vi "Get Tweets Search New.vi"(8 "error in":errorcluster, 9 "Tweets to Read (10)":i32=10 min=0 max=200 step=1, 10 "Query":string="#LVHacker", 11 "Twitter Handle In":T1={"OAuth Credentials"={"Signature Method"=enum."HMAC-SHA1", "Version"="1.0", "Client"={"Token"="", "Secret"=""}, "Access"={"Token"="", "Secret"=""}}, "since ID"="", "max ID"="", "Screen Name"=""}) -> (0 "error out":errorcluster, 1 "Actual Num of Tweets Read":i32, 2 "New Tweets Read":T5[](array[typedef]), 3 "Twitter Handle Out":T1={"OAuth Credentials"={"Signature Method"=enum."HMAC-SHA1", "Version"="1.0", "Client"={"Token"="", "Secret"=""}, "Access"={"Token"="", "Secret"=""}}, "since ID"="", "max ID"="", "Screen Name"=""}, 5 "Time Stamp of Newest Tweet":timestamp)   [LabVIEW 2011, in "i3-twitter.lvlib"]
doc: "Use this VI to search for Tweets based on a <b>Search Query</b>. A common Search Query may be a hashtag search such as #LVHacker. <b>Get Tweets Search New.vi</b> returns new Tweets for the authenticated user since the last time this function was called with the <b>Twitter Handle</b>.\n\nThe first time the function is called it returns the number of Tweets specified by <b>Tweets to Read</b> and each consecutive call returns Tweets that have been received after the <b>Time Stamp of Newest Tweet</b>."
uses:
  i3-twitter.lvlib
  Controls/Tweet.ctl
  Controls/Twitter Handle.ctl
  i3-oauth/Controls/OAuth Handle.ctl
  i3-oauth/Controls/Signature Method.ctl
  i3-oauth/Controls/Credentials.ctl
  i3-oauth/Controls/HTTP Method.ctl
  i3-json/JSON Parsing/Get Object Parameter Files/Get Object Parameter - Object.vi
  i3-json/JSON Parsing/Get Array Value at Index Files/Get Array Value at Index - Object.vi
  i3-json/JSON Parsing/Get Object Parameter Files/Get Object Parameter - String.vi
  i3-oauth/i3-oauth.lvlib
  <vilib>/httpClient/LabVIEWHTTPClient.lvlib
  i3-json/i3-json.lvlib
panel:
  out "Full URL":string
  out "body":string
  out "headers":string
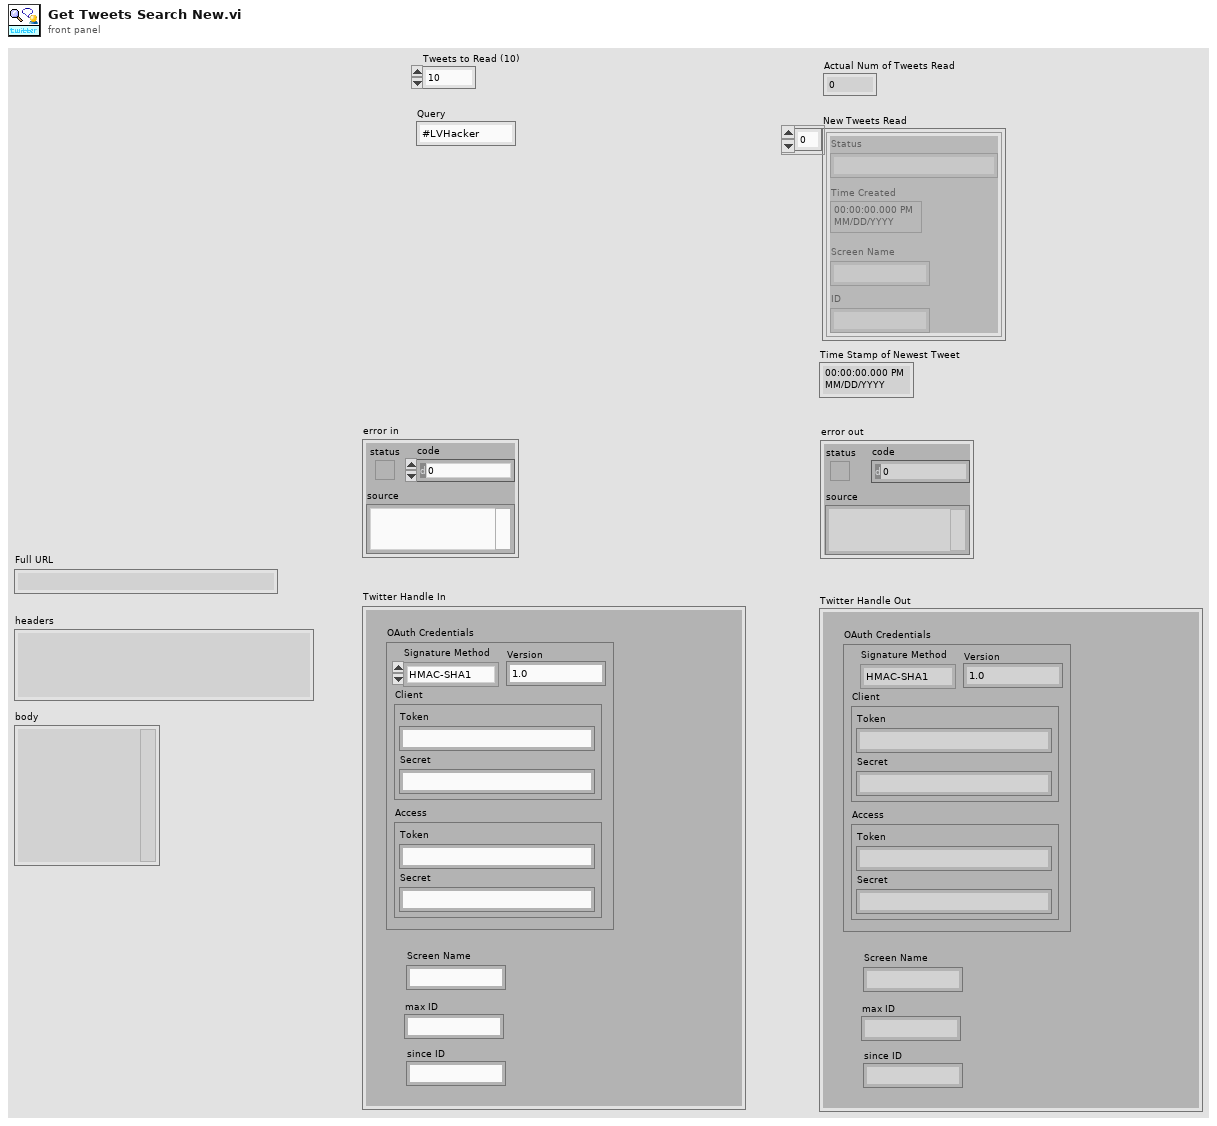
[diagram p1: front panel]
types:
  T1 = typedef "i3-twitter.lvlib/Twitter Handle.ctl" = cluster{"OAuth Credentials":T2, "since ID":string, "max ID":string, "Screen Name":string}
  T2 = typedef "i3-oauth.lvlib/OAuth Handle.ctl" = cluster{"Signature Method":T3, "Version":string, "Client":T4, "Access":T4}
  T3 = typedef "i3-oauth.lvlib/Signature Method.ctl" = enum16{"HMAC-MD5", "HMAC-SHA1", "HMAC-SHA224", "HMAC-SHA256", "HMAC-SHA384", "HMAC-SHA512"}
  T4 = typedef "i3-oauth.lvlib/Credentials.ctl" = cluster{"Token":string, "Secret":string}
  T5 = typedef "i3-twitter.lvlib/Tweet.ctl" = cluster{"Status":string, "Time Created":timestamp, "Screen Name":string, "ID":string}
  T6 = typedef "i3-oauth.lvlib/HTTP Method.ctl" = enum16{"GET", "POST", "PUT", "DELETE"}
  T7 = typedef "i3-oauth.lvlib/Name-Value Pair.ctl" = cluster{"Name":string, "Value":string}
  T8 = typedef "LabVIEWHTTPClient.lvlib/ClientHandle.ctl" = refnum<k1>
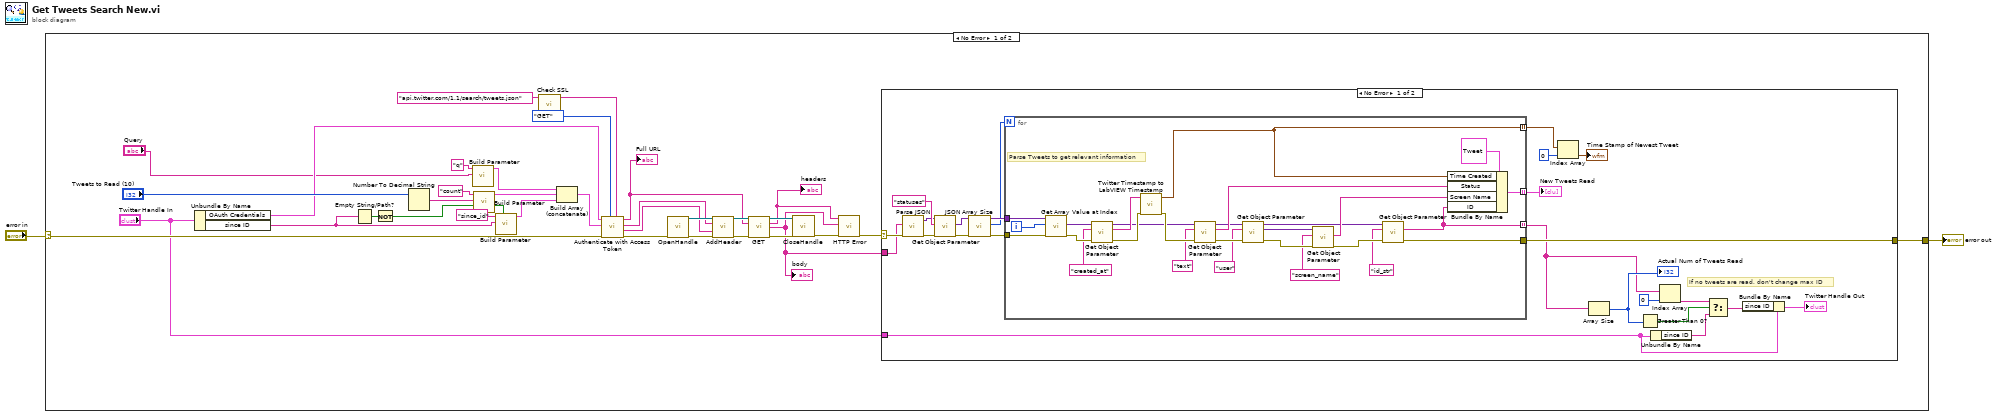
[diagram p0: block diagram]
diagram:
  n1 = case shown="No Error" "error in" {
    selector: "error in" -> [w36 w89]
    tunnel: [w18 w89] -> w2
    frame No Error {
      n2 = Unbundle By Name("Twitter Handle In") -> ("OAuth Credentials"=w15:T2, "since ID"=w5:string)
      n3 = Empty String/Path?(string/path=w5) -> (empty?=w6:bool)
      n4 = Not(x=w6) -> (.not. x?=w4:bool)
      n5 = Number To Decimal String(number="Tweets to Read (10)") -> (decimal integer string=w24:string)  [unwired: 1 in]
      n6 = call "Build Parameter.vi"("Value"="Query", "Key"="q") -> ("Parameter Array"=w9:T7[])  [unwired: 9 in]
      n7 = call "Build Parameter.vi"("Value"=w24, "Key"="count") -> ("Parameter Array"=w12:T7[])  [unwired: 9 in]
      n8 = call "Build Parameter.vi"("Return Parameter? (T)"=w4, "Value"=w5, "Key"="since_id") -> ("Parameter Array"=w3:T7[])  [unwired: 8 in]
      n9 = call "Check SSL.vi"("Input URL"="api.twitter.com/1.1/search/tweets.json" ("Base URL")) -> ("Output URL"=w13:string)  [unwired: 8 in]
      n10 = Build Array (concatenate)(w9, w12, w3) -> (w23:T7[])
      n11 = call "Authenticate with Access Token.vi"("Base URL"=w13, "HTTP Method"=HTTP_Method."GET", "error in (no error)"=w36, "URL Parameters"=w23, "OAuth Handle"=w15) -> ("error out"=w22:errorcluster, "Header Value"=w28:string, "Header Parameter"=w29:string, "Full URL"=w27:string)  [unwired: 2 in, 1 out]
      "Full URL" <- w27
      n12 = call <vilib>:"OpenHandle.vi"("error in (no error)"=w22) -> ("client handle out"=w35:T8, "error out"=w34:errorcluster)  [unwired: 13 in]
      n13 = call <vilib>:"AddHeader.vi"("client handle"=w35, "header"=w29, "value"=w28, "error in (no error)"=w34) -> ("client handle out"=w33:T8, "error out"=w32:errorcluster)  [unwired: 10 in]
      n14 = call <vilib>:"GET.vi"("client handle"=w33, "url"=w27, "error in (no error)"=w32) -> ("client handle out"=w31:T8, "headers"=w21:string, "body"=w17:string, "error out"=w30:errorcluster)  [unwired: 9 in]
      "body" <- w17
      "headers" <- w21
      n15 = call <vilib>:"CloseHandle.vi"("client handle"=w31, "error in (no error)"=w30) -> ("error out"=w20:errorcluster)  [unwired: 13 in]
      n16 = call "HTTP Error.vi"("error in (no error)"=w20, "Body"=w17, "Header"=w21) -> ("error out"=w19:errorcluster)  [unwired: 6 in, 2 out]
      n17 = case shown="No Error" w19 {
        selector: w19 -> [w56 w88]
        tunnel: [w55 w88] -> w18
        tunnel: w17 -> [w54 _]
        tunnel: "Twitter Handle In" -> [w37 _]
        frame No Error {
          # "If no tweets are read, don't change max ID"
          n18 = call "Parse JSON.vi"("error in (no error)"=w56, "JSON String"=w54) -> ("error out"=w46:errorcluster, "JSON Tree"=w47:variant)  [unwired: 6 in, 2 out]
          n19 = call-poly "Get Object Parameter.vi"("error in (no error)"=w46, "Parameter Name"="statuses", "JSON Tree In (JSON Object)"=w47) -> ("error out"=w50:errorcluster, "JSON Object"=w49:variant)  [unwired: 5 in, 2 out]
          n20 = call "JSON Array Size.vi"("error in (no error)"=w50, "JSON Tree In (JSON Array)"=w49) -> ("error out"=w58:errorcluster, "Array Size"=w59:i32, "JSON Tree Passthrough (JSON Array)"=w60:variant)  [unwired: 7 in]
          n21 = for {
            N: w59 -> [_]
            tunnel: w58 -> [w71]
            tunnel: [w74] -> w57 mode=indexing
            tunnel: [w73] -> w55
            tunnel: w60 -> [w70]
            tunnel: [w69] -> w53 mode=indexing
            tunnel: [w61] -> w38 mode=indexing
            i -> [w76]
            # "Parse Tweets to get relevant information"
            n22 = call-poly "Get Array Value at Index.vi"("error in (no error)"=w71, "Index"=w76, "JSON Tree In (JSON Array)"=w70) -> ("error out"=w83:errorcluster, "JSON Object"=w67:variant)  [unwired: 5 in, 2 out]
            n23 = call-poly "Get Object Parameter.vi"("error in (no error)"=w83, "Parameter Name"="created_at", "JSON Tree In (JSON Object)"=w67) -> ("error out"=w66:errorcluster, "String Value"=w65:string, "JSON Tree Out Passthrough"=w64:variant)  [unwired: 5 in, 1 out]
            n24 = call "Twitter Timestamp to LabVIEW Timestamp.vi"("error in"=w66, "Twitter Time Stamp"=w65) -> ("error out"=w84:errorcluster, "LabVIEW Time Stamp"=w69:timestamp)  [unwired: 6 in]
            n25 = call-poly "Get Object Parameter.vi"("error in (no error)"=w84, "Parameter Name"="text", "JSON Tree In (JSON Object)"=w64) -> ("error out"=w85:errorcluster, "String Value"=w72:string, "JSON Tree Out Passthrough"=w63:variant)  [unwired: 5 in, 1 out]
            n26 = call-poly "Get Object Parameter.vi"("error in (no error)"=w85, "Parameter Name"="user", "JSON Tree In (JSON Object)"=w63) -> ("error out"=w86:errorcluster, "JSON Object"=w68:variant, "JSON Tree Out Passthrough"=w62:variant)  [unwired: 5 in, 1 out]
            n27 = call-poly "Get Object Parameter.vi"("error in (no error)"=w86, "Parameter Name"="screen_name", "JSON Tree In (JSON Object)"=w68) -> ("error out"=w87:errorcluster, "String Value"=w79:string)  [unwired: 5 in, 2 out]
            n28 = call-poly "Get Object Parameter.vi"("error in (no error)"=w87, "Parameter Name"="id_str", "JSON Tree In (JSON Object)"=w62) -> ("error out"=w73:errorcluster, "String Value"=w61:string)  [unwired: 5 in, 2 out]
            n29 = Bundle By Name(cluster=T5 {"Status"="", "Time Created"=timestamp(0 s since 1904-01-01), "Screen Name"="", "ID"=""}, "Time Created"=w69, "Status"=w72, "Screen Name"=w79, "ID"=w61) -> (w74:T5)
          }
          "New Tweets Read" <- w57
          n30 = Index Array(array=w53, index=0) -> (element=→"Time Stamp of Newest Tweet":timestamp)
          n31 = Array Size(array=w38) -> (size(s)=w44:i32)
          "Actual Num of Tweets Read" <- w44
          n32 = Greater Than 0?(x=w44) -> (x > 0?=w45:bool)
          n33 = Unbundle By Name(w37) -> ("since ID"=w39:string)
          n34 = Index Array(array=w38, index=0) -> (element=w43:string)
          n35 = Select(t=w43, s=w45, f=w39) -> (s? t:f=w42:string)
          n36 = Bundle By Name(cluster=w37, "since ID"=w42) -> (→"Twitter Handle Out":T1)
        }
        frame Error {
        }
      }
    }
    frame Error {
    }
  }
  "error out" <- w2
